vi "S2C_ExeGetLoopRef.vi"(8 "Error In":errorcluster) -> (0 "Error Out":errorcluster)   [LabVIEW 2015]
uses:
  Globals/S2C_Globals.vi
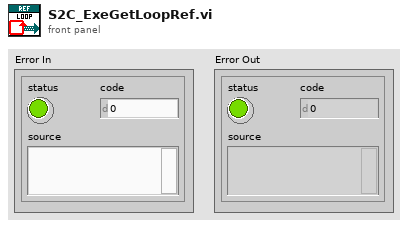
[diagram p1: front panel]
types:
  T1 = cluster{"Foreground Color":u32, "Background Color":u32}
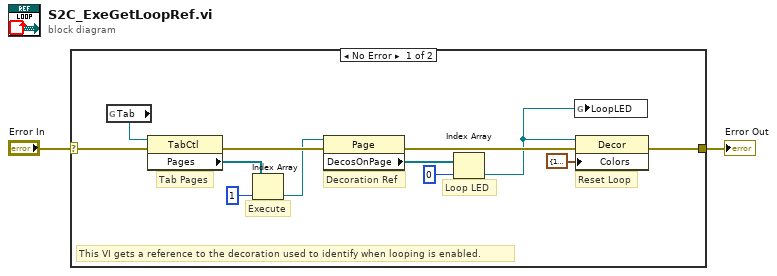
[diagram p0: block diagram]
diagram:
  n1 = case shown="No Error" "Error In" {
    selector: "Error In" -> [w14 w15]
    tunnel: [w8 w15] -> w1
    frame No Error {
      # "This VI gets a reference to the decoration used to identify when looping is enabled."
      # "Loop LED"
      # "Execute"
      # "Reset Loop"
      # "Decoration Ref"
      # "Tab Pages"
      n2 = global read "S2C_Globals.vi" "Tab"() -> (w13:refnum<vi>)
      n3 = property class="TabCtl"(reference=w13, error in=w14) -> (error out=w12:errorcluster, "Pages"=w5:refnum<vi>[])  [unwired: 1 out]
      n4 = Index Array(array=w5, index=1) -> (element=w4:refnum<vi>)
      n5 = property class="Page"(reference=w4, error in=w12) -> (error out=w11:errorcluster, "DecosOnPage"=w7:refnum<vi>[])  [unwired: 1 out]
      n6 = Index Array(array=w7, index=0) -> (element=w10:refnum<vi>)
      n7 = global write "S2C_Globals.vi" "LoopLED"(w10) -> ()
      n8 = property class="Decor"(reference=w10, error in=w11, "Colors"=T1 {"Foreground Color"=16777216, "Background Color"=16777216} ("Trans")) -> (error out=w8:errorcluster)  [unwired: 1 out]
    }
    frame Error {
    }
  }
  "Error Out" <- w1
